vi "Stop Process.vi"(8 "error in":errorcluster, 11 "tcp server in":refnum<class "RT FlexRIO Server TCP.lvclass">) -> (0 "error out":errorcluster, 3 "tcp server out":refnum<class "RT FlexRIO Server TCP.lvclass">)   [LabVIEW 2017, in "RT FlexRIO Server TCP.lvclass"]
uses:
  RT FlexRIO Server TCP.lvclass
  RT FlexRIO Server TCP.lvclass/RT FlexRIO Server TCP.ctl
  State.ctl
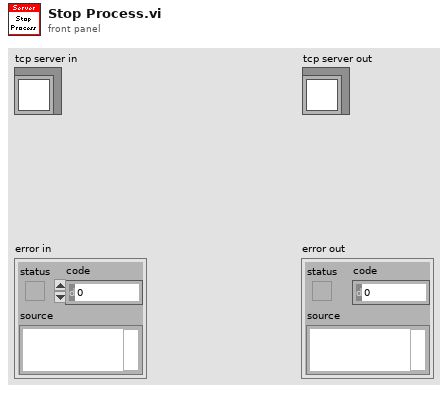
[diagram p1: front panel]
types:
  T1 = typedef "RT FlexRIO Server TCP.lvclass/SessionData.ctl" = cluster{"listener":refnum<k5>, "connection":refnum<k5>, "state":T2, "incoming":refnum<queue>, "outgoing":refnum<queue>, "state request":refnum<user-event>, "state changed":refnum<user-event>}
  T2 = typedef "RT FlexRIO Server TCP.lvclass/connection state.ctl" = enum16{"started", "connected", "stopped"}
  T3 = typedef "RT FlexRIO Server TCP.lvclass/State.ctl" = enum16{"started", "connected", "stopped"}
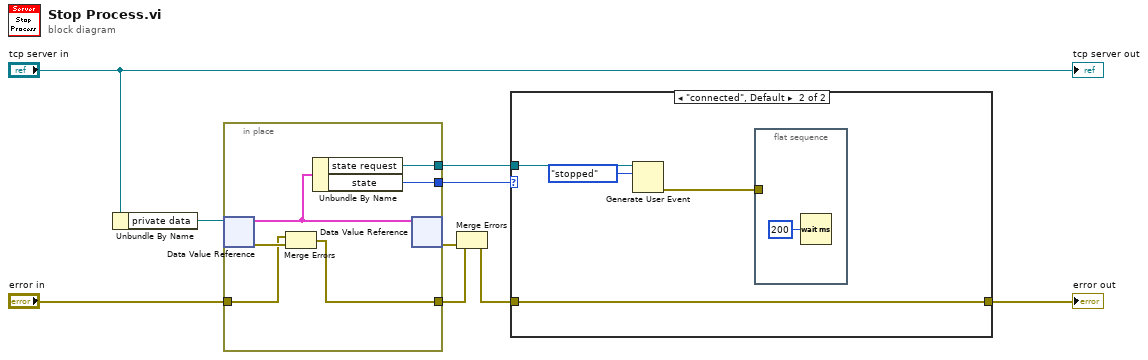
[diagram p0: block diagram]
diagram:
  n1 = Unbundle By Name("tcp server in") -> ("private data"=w9:refnum<data-value>)
  n2 = in-place {
    in-place-border: "error in" -> [w11]
    in-place-border: [w15] -> w7
    in-place-border: [w13] -> w5
    in-place-border: [w10] -> w3
    n3 = in-place-dvr #1(w9) -> (w14:T1, w12:errorcluster)
    n4 = Merge Errors(w11, w12) -> (w15:errorcluster)
    n5 = Unbundle By Name(w14) -> ("state request"=w13:refnum<user-event>, "state"=w10:T2)
    n6 = in-place-dvr #1(w14) -> (w8:errorcluster)  [unwired: 1 out]
  }
  n7 = Merge Errors(w7, w8) -> (w1:errorcluster)
  n8 = case shown="\"connected\", Default" w3 {
    tunnel: w5 -> [_ w20]
    tunnel: [w16 w18] -> w2
    tunnel: w1 -> [w16 w18]
    frame "stopped" {
    }
    frame "connected", Default {
      n9 = Generate User Event(user event=w20, event data cluster=State."stopped" ("connection state")) -> (error out=w17:errorcluster)  [unwired: 2 in, 1 out]
      n10 = flat-sequence {
        tunnel: w17 -> [_]
        frame #0 {
          n11 = Wait (ms)(milliseconds to wait=u32 200) -> ()  [unwired: 1 out]
        }
      }
    }
  }
  "error out" <- w2
  "tcp server out" <- "tcp server in"
